vi "Charact One Standard.vi"(0 "Vector Path in":refnum<class "Vector 18GHz Path.lvclass">, 5 "Standard Type":T2, 11 "error in":errorcluster) -> (4 "Vector Path out":refnum<class "Vector 18GHz Path.lvclass">, 6 "One-Port Charact Data":T1, 15 "error out":errorcluster)   [LabVIEW 2023, in "RFFixtureCharact.RFPM.lvlib" / "Vector 18GHz Path.lvclass"]
uses:
  Vector 18GHz Path.lvclass
  Instruments/Cal Standard/Type Definitions/Standard Type.ctl
  Instruments/Cal Standard/Type Definitions/One-Port Charact Data.ctl
  <instrlib>/niRFPM/niRFPM.llb/NI-RFPM Fetch S-Parameter Measurements Complex.vi
  Instruments/Cal Standard/Cal Standard Base/Cal Standard Base.lvclass
  Instruments/RFFixtureCharact.Instruments.lvlib
  Instruments/Cal Standard/Cal Standard Factory/Cal Standard Factory.lvclass
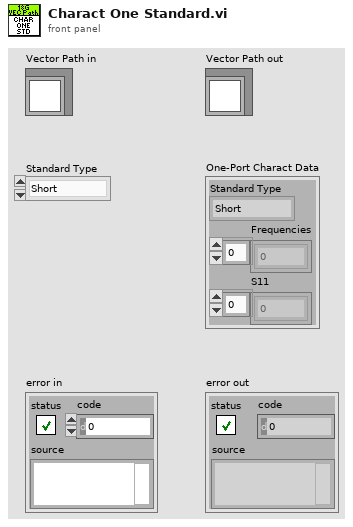
[diagram p1: front panel]
types:
  T1 = typedef "RFFixtureCharact.Instruments.lvlib/One-Port Charact Data.ctl" = cluster{"Standard Type":T2, "Frequencies":dbl[], "S11":cdb[]}
  T2 = typedef "RFFixtureCharact.Instruments.lvlib/Standard Type.ctl" = enum16{"Short", "Open", "Load", "PowerMeter", "None"}
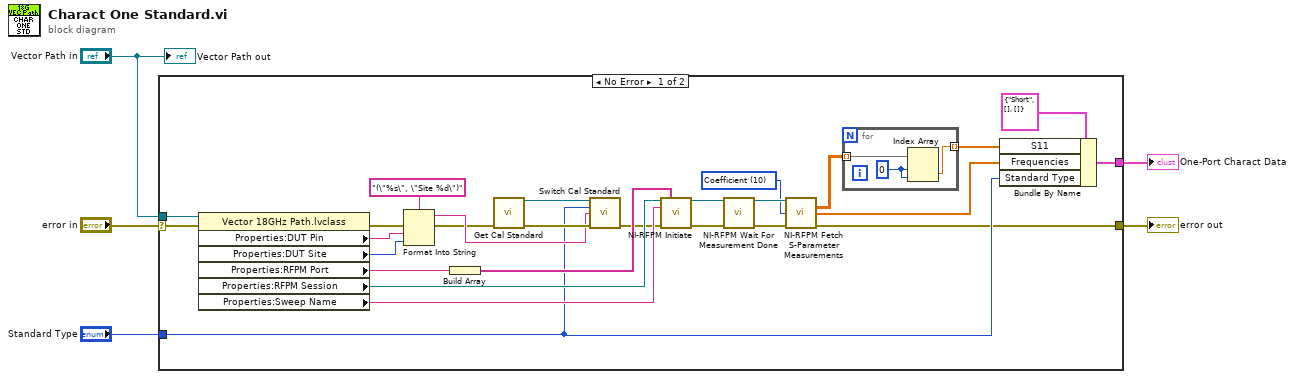
[diagram p0: block diagram]
diagram:
  n1 = case shown="No Error" "error in" {
    selector: "error in" -> [w29 w36]
    tunnel: [w6 w36] -> w3
    tunnel: "Vector Path in" -> [w32 _]
    tunnel: "Standard Type" -> [w10 _]
    tunnel: [w7 _] -> w1
    frame No Error {
      w17 = 10 items=["Coefficient"=10] ("format")
      n2 = property on="Property Node" class="Vector 18GHz Path.lvclass"(reference=w32, error in=w29) -> (error out=w8:errorcluster, "Properties:DUT Pin"=w9:string, "Properties:DUT Site"=w23:i32, "Properties:RFPM Port"=w28:string, "Properties:RFPM Session"=w20:refnum<k15>, "Properties:Sweep Name"=w30:string)  [unwired: 1 out]
      n3 = Format Into String(format string="(\"%s\", \"Site %d\")", error in=w8, w9, w23) -> (resulting string=w22:string, error out=w21:errorcluster)  [unwired: 1 in]
      n4 = Build Array(w28) -> (w31:string[])
      n5 = call "Get Cal Standard.vi"("error in (no error)"=w21) -> ("Cal Standard Base out"=w25:refnum<class "Cal Standard Base.lvclass">, "error out"=w26:errorcluster)  [unwired: 12 in, 1 out]
      n6 = call-dynamic "Switch Cal Standard.vi"("Cal Standard Base in"=w25, "Standard Type"=w10, "Path Name"=w22, "error in (no error)"=w26) -> ("error out"=w11:errorcluster)  [unwired: 10 in, 1 out]
      n7 = call <instrlib>:"NI-RFPM Initiate.vi"("instrument handle"=w20, "Ports"=w31, "Sweep Setting Name"=w30, "error in"=w11) -> ("instrument handle out"=w12:refnum<k15>, "error out"=w13:errorcluster)  [unwired: 10 in]
      n8 = call <instrlib>:"NI-RFPM Wait For Measurement Done.vi"("instrument handle"=w12, "error in"=w13) -> ("instrument handle out"=w19:refnum<k15>, "error out"=w18:errorcluster)  [unwired: 12 in]
      n9 = call-poly <instrlib>:"NI-RFPM Fetch S-Parameter Measurements.vi"("instrument handle"=w19, "format"=w17, "error in"=w18) -> ("data"=w16:cdb[][][], "frequency"=w27:dbl[], "error out"=w6:errorcluster)  [unwired: 8 in, 2 out]
      n10 = for {
        tunnel: w16 -> [w35] mode=indexing
        tunnel: [w34] -> w15 mode=indexing
        w33 = 0 ("index (row)")
        n11 = Index Array(array=w35, index (row)=w33, index (col)=w33) -> (element=w34:cdb)
      }
      n12 = Bundle By Name(cluster=T1 {"Standard Type"=enum."Short", "Frequencies"=[], "S11"=[]} ("One-Port Charact Data"), "S11"=w15, "Frequencies"=w27, "Standard Type"=w10) -> (w7:T1)
    }
    frame Error {
    }
  }
  "error out" <- w3
  "One-Port Charact Data" <- w1
  "Vector Path out" <- "Vector Path in"
